vi "GET_Initial_Conditions_representation_2.vi"(2 "error in (no error)":errorcluster, 3 "Input parameters cluster":T1 {"Calibration parameters"."True frame time, s" format="%.10g"; "Calibration parameters"."Disp. calibration info"."Speed, µl per ms" format="%.3g"; "Calibration parameters"."True FPS" format="%.10g"; "Calibration parameters"."Timing calibration sw/hw" format="%.10g"}) -> (0 "error out":errorcluster)   [LabVIEW 2018, in "Tracker.lvlib"]
uses:
  Tracker.lvlib
  Controls/CTL_Conditions_build_parameters_2.ctl
  Classes/Reward_Condition/Controls/RC_Array_of_Conditions.ctl
  Classes/Reward_Condition/Reward_Condition.lvclass
  Controls/CTL_Calibration_parameters.ctl
  Controls/CTL_Dispenser_calibration_info.ctl
  Common_Resources.lvlib
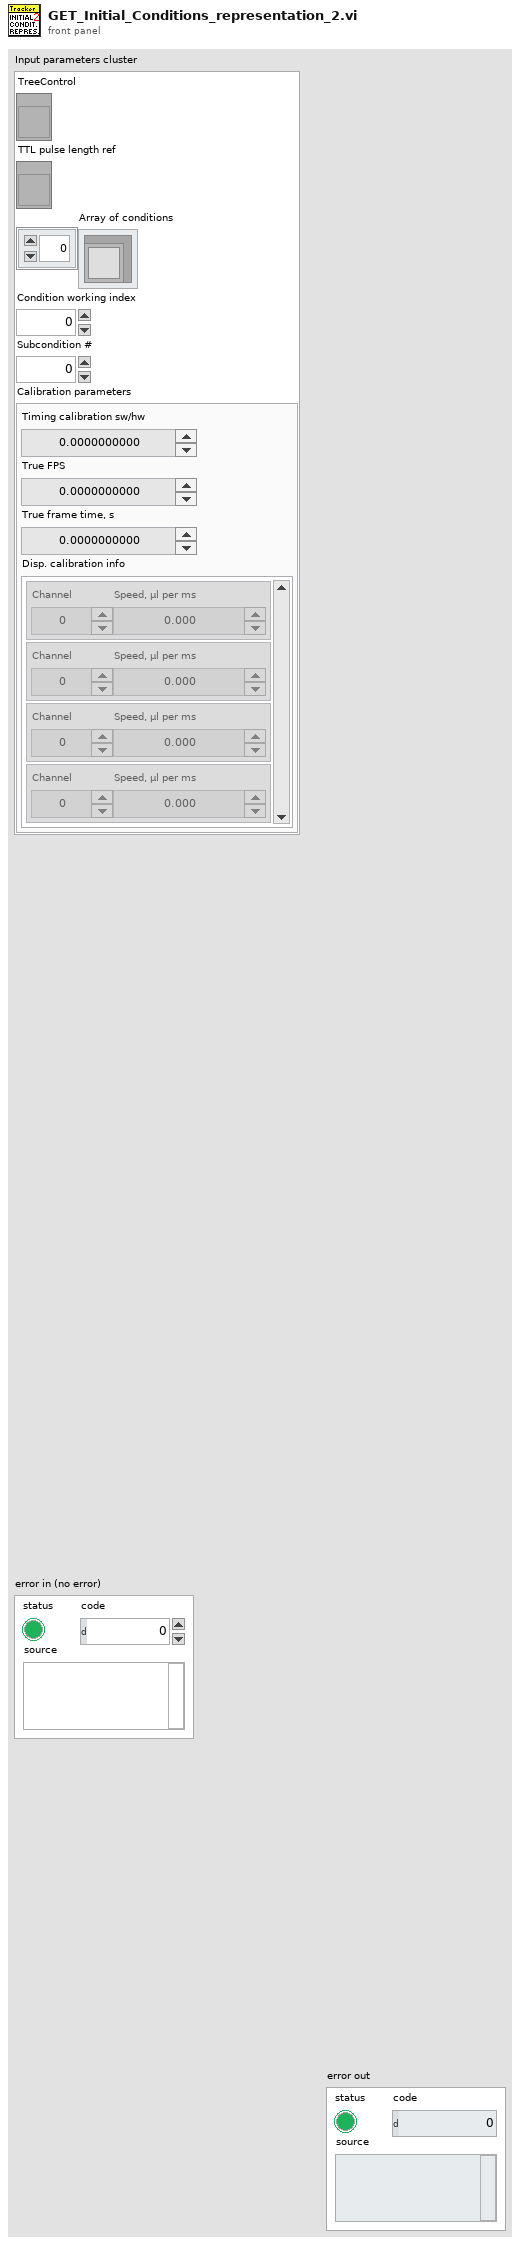
[diagram p1: front panel]
types:
  T1 = typedef "Common_Resources.lvlib/CTL_Conditions_build_parameters_2.ctl" = cluster{"TreeControl":refnum<vi>, "TTL pulse length ref":refnum<vi>, "Array of conditions":T2, "Condition working index":i32, "Subcondition #":i32, "Calibration parameters":T3}
  T2 = typedef "Tracker.lvlib/Reward_Condition.lvclass/RC_Array_of_Conditions.ctl" = refnum<class "Reward_Condition.lvclass">[]
  T3 = typedef "Common_Resources.lvlib/CTL_Calibration_parameters.ctl" = cluster{"Timing calibration sw/hw":dbl, "True FPS":dbl, "True frame time, s":dbl, "Disp. calibration info":T4}
  T4 = typedef "Common_Resources.lvlib/CTL_Dispenser_calibration_info.ctl" = cluster{"Channel":u8, "Speed, µl per ms":dbl}[]
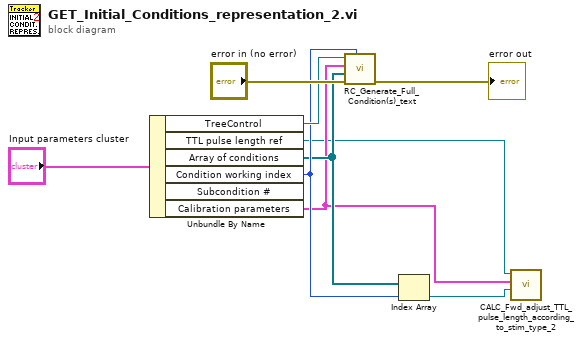
[diagram p0: block diagram]
diagram:
  n1 = Unbundle By Name("Input parameters cluster") -> ("TreeControl"=w6:refnum<vi>, "TTL pulse length ref"=w1:refnum<vi>, "Array of conditions"=w4:T2, "Condition working index"=w5:i32, "Calibration parameters"=w3:T3)  [unwired: 1 out]
  n2 = call "RC_Generate_Full_Condition(s)_text.vi"("Array index to show"=w5, "error in (no error)"="error in (no error)", "Array of conditions in"=w4, "Calibration parameters"=w3, "TreeControl ref in"=w6) -> ("error out"=→"error out":errorcluster)  [unwired: 5 in, 1 out]
  n3 = Index Array(array=w4, index=w5) -> (element=w2:refnum<class "Reward_Condition.lvclass">)
  n4 = call "CALC_Fwd_adjust_TTL_pulse_length_according_to_stim_type_2.vi"("Condition"=w2, "Calibration parameters"=w3, "TTL pulse length ref in"=w1) -> ()  [unwired: 9 in]
